vi "_ConnectorPaneEditor_ActiveShortcutMenu.vi"(8 "error in (no error)":errorcluster, 9 "MenuRef":refnum<k9>, 10 "CPpictureRef":refnum<vi>, 11 "ConnectorPaneEditor in":refnum<class "_ConnectorPaneEditor.lvclass">) -> (0 "error out":errorcluster, 3 "ConnectorPaneEditor out":refnum<class "_ConnectorPaneEditor.lvclass">)   [LabVIEW 2014, in "_ConnectorPaneEditor.lvclass"]
uses:
  _ConnectorPaneEditor.lvclass
  _ConnectorPaneEditor.lvclass/_ConnectorPaneEditor.ctl
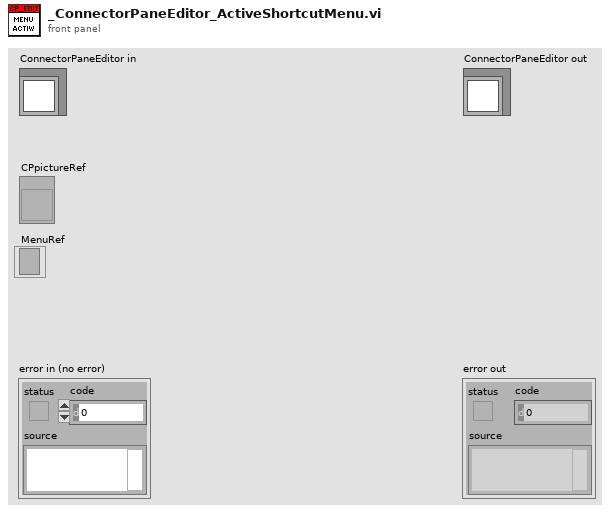
[diagram p1: front panel]
types:
  T1 = typedef "LVRectTypeDef.ctl" = cluster{"Left":i16, "Top":i16, "Right":i16, "Bottom":i16}
  T2 = typedef "LVMouseTypeDef.ctl" = cluster{"Mouse Position":cluster{"X":i32, "Y":i32}, "Mouse Modifiers":cluster{"Button Down":bool, "Shift Mod":bool, "Menu Mod":bool, "Option Mod":bool}}
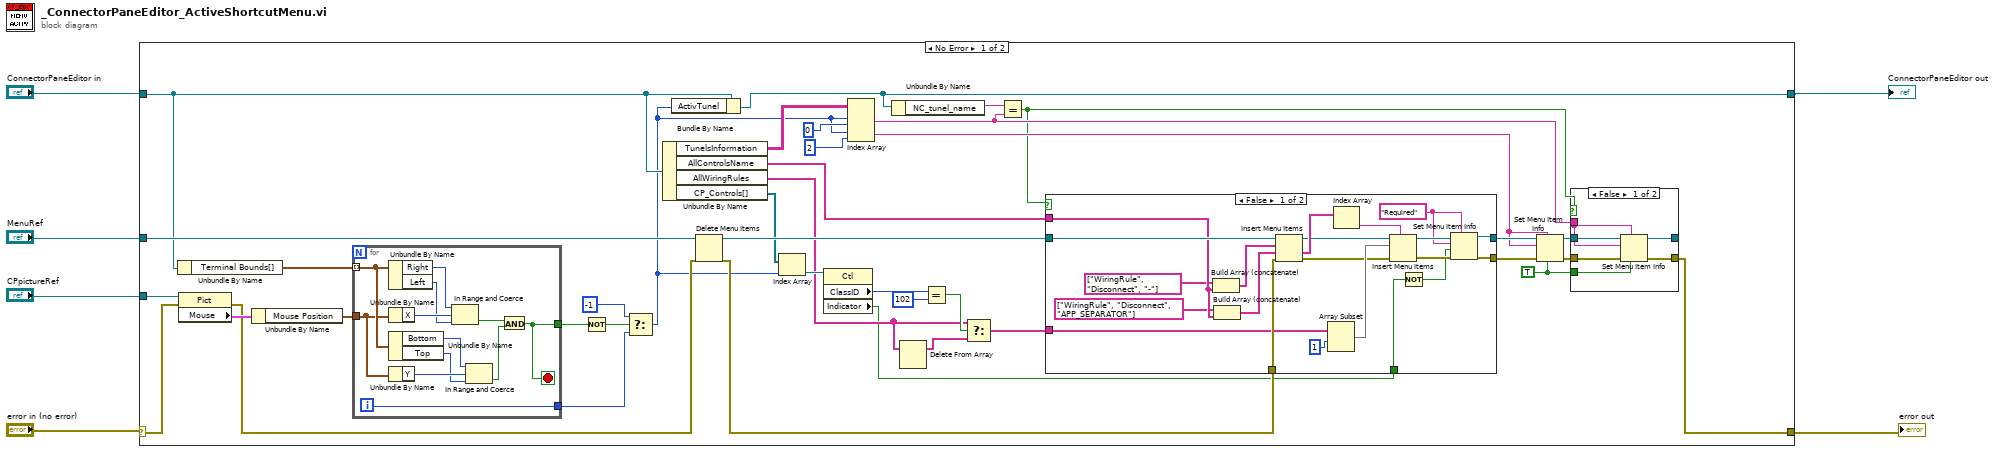
[diagram p0: block diagram]
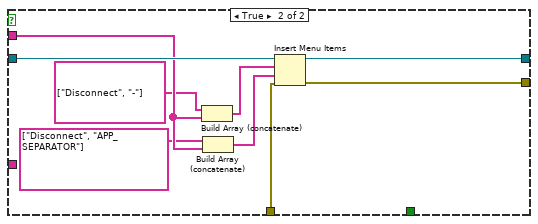
[diagram p2: hidden frame]
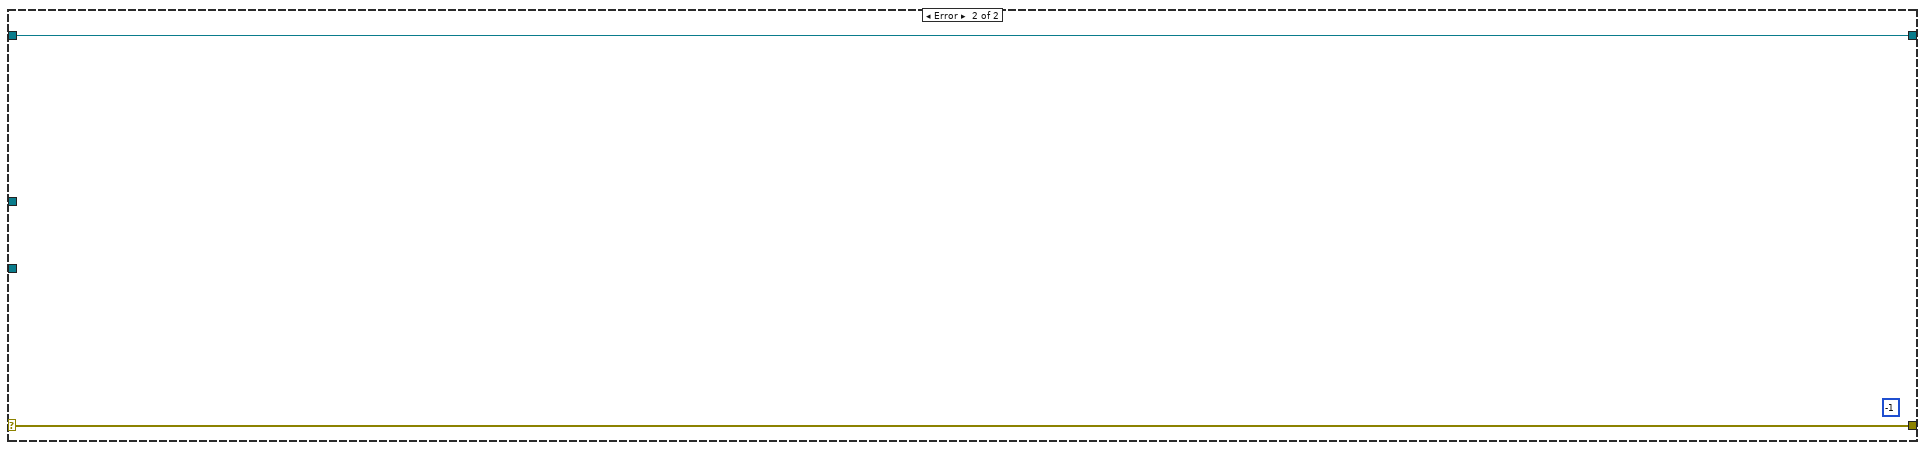
[diagram p4: hidden frame]
diagram:
  n1 = case shown="No Error" "error in (no error)" {
    selector: "error in (no error)" -> [w44 w97]
    tunnel: [w8 w97] -> w4
    tunnel: [w22 w96] -> w3
    tunnel: "ConnectorPaneEditor in" -> [w23 w96]
    tunnel: "CPpictureRef" -> [w37 _]
    tunnel: "MenuRef" -> [w33 _]
    frame No Error {
      w25 = TRUE ("checked")
      n2 = Unbundle By Name(w23) -> ("Terminal Bounds[]"=w38:T1[])
      n3 = property class="Pict"(reference=w37, error in=w44) -> (error out=w32:errorcluster, "Mouse"=w45:T2)  [unwired: 1 out]
      n4 = Unbundle By Name(w45) -> ("Mouse Position"=w43:cluster{"X":i32, "Y":i32})
      n5 = for {
        tunnel: w38 -> [w92] mode=indexing
        tunnel: w43 -> [w91]
        tunnel: [w85] -> w40
        tunnel: [w84] -> w42
        i -> [w85]
        stop <- w84 stop-if-true
        n6 = Unbundle By Name(w92) -> ("Right"=w94:i16, "Left"=w93:i16)
        n7 = Unbundle By Name(w91) -> ("X"=w95:i32)
        n8 = Unbundle By Name(w92) -> ("Bottom"=w89:i16, "Top"=w88:i16)
        n9 = Unbundle By Name(w91) -> ("Y"=w90:i32)
        n10 = In Range and Coerce(upper limit=w94, x=w95, lower limit=w93) -> (In Range?=w87:bool)  [unwired: 1 out]
        n11 = In Range and Coerce(upper limit=w89, x=w90, lower limit=w88) -> (In Range?=w86:bool)  [unwired: 1 out]
        n12 = And(x=w87, y=w86) -> (x .and. y?=w84:bool)
      }
      n13 = Not(x=w42) -> (.not. x?=w41:bool)
      n14 = Select(t=-1, s=w41, f=w40) -> (s? t:f=w16:i32)
      n15 = Unbundle By Name(w23) -> ("TunelsInformation"=w34:string[][], "AllControlsName"=w19:string[], "AllWiringRules"=w10:string[], "CP_Controls[]"=w17:refnum<vi>[])
      n16 = Bundle By Name(cluster=w23, "ActivTunel"=w16) -> (w22:refnum<class "_ConnectorPaneEditor.lvclass">)
      n17 = Delete Menu Items(6:w32, 9:w33) -> (0:w30:errorcluster, 3:w31:refnum<k9>)  [unwired: 2 in]
      n18 = Index Array(array=w17, index=w16) -> (element=w15:refnum<vi>)
      n19 = property class="Ctl"(reference=w15) -> ("ClassID"=w14:u32, "Indicator"=w7:bool)  [unwired: 1 in, 2 out]
      n20 = Index Array(array=w34, index (row) #1=w16, index (col) #1=0 ("disabled index (col)"), index (row) #2=w16, index (col) #2=2 ("index (col)")) -> (element #1=w20:string, element #2=w24:string)
      n21 = Unbundle By Name(w22) -> ("NC_tunel_name"=w21:string)
      n22 = Delete From Array(array=w10) -> (array with subset deleted=w9:string[])  [unwired: 2 in, 1 out]
      n23 = Equal?(x=w14, y=u32 102) -> (x = y?=w12:bool)
      n24 = Select(t=w10, s=w12, f=w9) -> (s? t:f=w11:string[])
      n25 = Equal?(x=w21, y=w20) -> (x = y?=w18:bool)
      n26 = case shown="False" w18 {
        tunnel: w31 -> [w66 w75]
        tunnel: w30 -> [w65 w74]
        tunnel: [w52 w67] -> w29
        tunnel: [w49 w68] -> w28
        tunnel: w19 -> [w56 w71]
        tunnel: w11 -> [w54 _]
        tunnel: w7 -> [w46 _]
        frame False {
          w48 = "Required" ("item tag")
          n27 = Build Array (concatenate)(string[] ["WiringRule", "Disconnect", "-"], w56) -> (w63:string[])
          n28 = Build Array (concatenate)(string[] ["WiringRule", "Disconnect", "APP_SEPARATOR"], w56) -> (w64:string[])
          n29 = Insert Menu Items(6:w65, 7:w64, 8:w63, 9:w66) -> (0:w57:errorcluster, 1:w62:string[], 3:w61:refnum<k9>)  [unwired: 2 in]
          n30 = Array Subset(array=w54, index=1) -> (w59:string[])  [unwired: 1 in]
          n31 = Index Array(array=w62) -> (element=w58:string)  [unwired: 1 in]
          n32 = Insert Menu Items(5:w58, 6:w57, 8:w59, 9:w61) -> (0:w51:errorcluster, 3:w50:refnum<k9>)  [unwired: 2 in, 1 out]
          n33 = Not(x=w46) -> (.not. x?=w47:bool)
          n34 = Set Menu Item Info(7:w48, 8:w51, 9:w47, 10:w48, 11:w50) -> (0:w52:errorcluster, 3:w49:refnum<k9>)  [unwired: 2 in]
        }
        frame True {
          n35 = Build Array (concatenate)(string[] ["Disconnect", "-"], w71) -> (w72:string[])
          n36 = Build Array (concatenate)(string[] ["Disconnect", "APP_SEPARATOR"], w71) -> (w73:string[])
          n37 = Insert Menu Items(6:w74, 7:w73, 8:w72, 9:w75) -> (0:w67:errorcluster, 3:w68:refnum<k9>)  [unwired: 2 in, 1 out]
        }
      }
      n38 = Set Menu Item Info(6:w25, 7:w24, 8:w29, 10:w24, 11:w28) -> (0:w27:errorcluster, 3:w26:refnum<k9>)  [unwired: 2 in]
      n39 = case shown="False" w18 {
        tunnel: w27 -> [w81 w83]
        tunnel: w26 -> [w80 w82]
        tunnel: w25 -> [w79 _]
        tunnel: w20 -> [w78 _]
        tunnel: [w77 w83] -> w8
        tunnel: [w76 w82] -> _
        frame False {
          n40 = Set Menu Item Info(6:w79, 7:w78, 8:w81, 10:w78, 11:w80) -> (0:w77:errorcluster, 3:w76:refnum<k9>)  [unwired: 2 in]
        }
        frame True {
        }
      }
    }
    frame Error {
      (unwired) -1
    }
  }
  "error out" <- w4
  "ConnectorPaneEditor out" <- w3
